vi "第一段判定.vi"(7 "Result":refnum<vi>, 10 "最大值判定":T1, 11 "XY曲线":cluster{"X":dbl[], "Y":dbl[]}[](array[cluster])) -> (2 "大小":i32, 3 "OK？":bool)   [LabVIEW 2020]
uses:
  Global_Variable/Global.vi
panel:
  in  "判定参数":T2
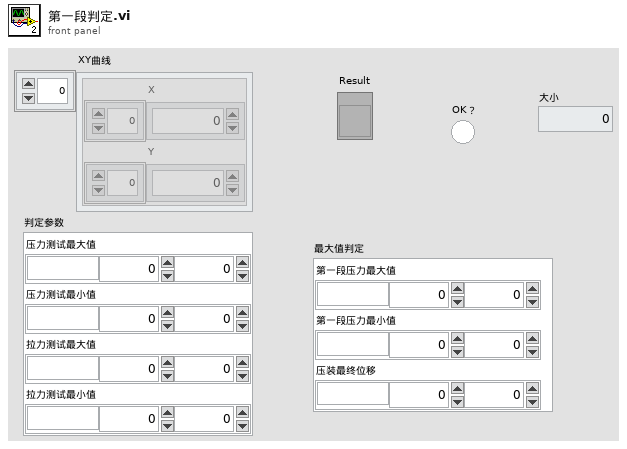
[diagram p1: front panel]
types:
  T1 = cluster{"第一段压力最大值":cluster{"单位":string, "下限":dbl, "上限":dbl}, "第一段压力最小值":cluster{"单位":string, "下限":dbl, "上限":dbl}, "压装最终位移":cluster{"单位":string, "下限":dbl, "上限":dbl}}
  T2 = cluster{"压力测试最大值":cluster{"单位":string, "下限":dbl, "上限":dbl}, "压力测试最小值":cluster{"单位":string, "下限":dbl, "上限":dbl}, "拉力测试最大值":cluster{"单位":string, "下限":dbl, "上限":dbl}, "拉力测试最小值":cluster{"单位":string, "下限":dbl, "上限":dbl}}
  T3 = cluster{"第一段判定框位移":cluster{"单位":string, "下限":dbl, "上限":dbl}, "第一段判定框压力":cluster{"单位":string, "下限":dbl, "上限":dbl}, "低二段判定框位移":cluster{"单位":string, "下限":dbl, "上限":dbl}, "第二段判定框压力":cluster{"单位":string, "下限":dbl, "上限":dbl}}
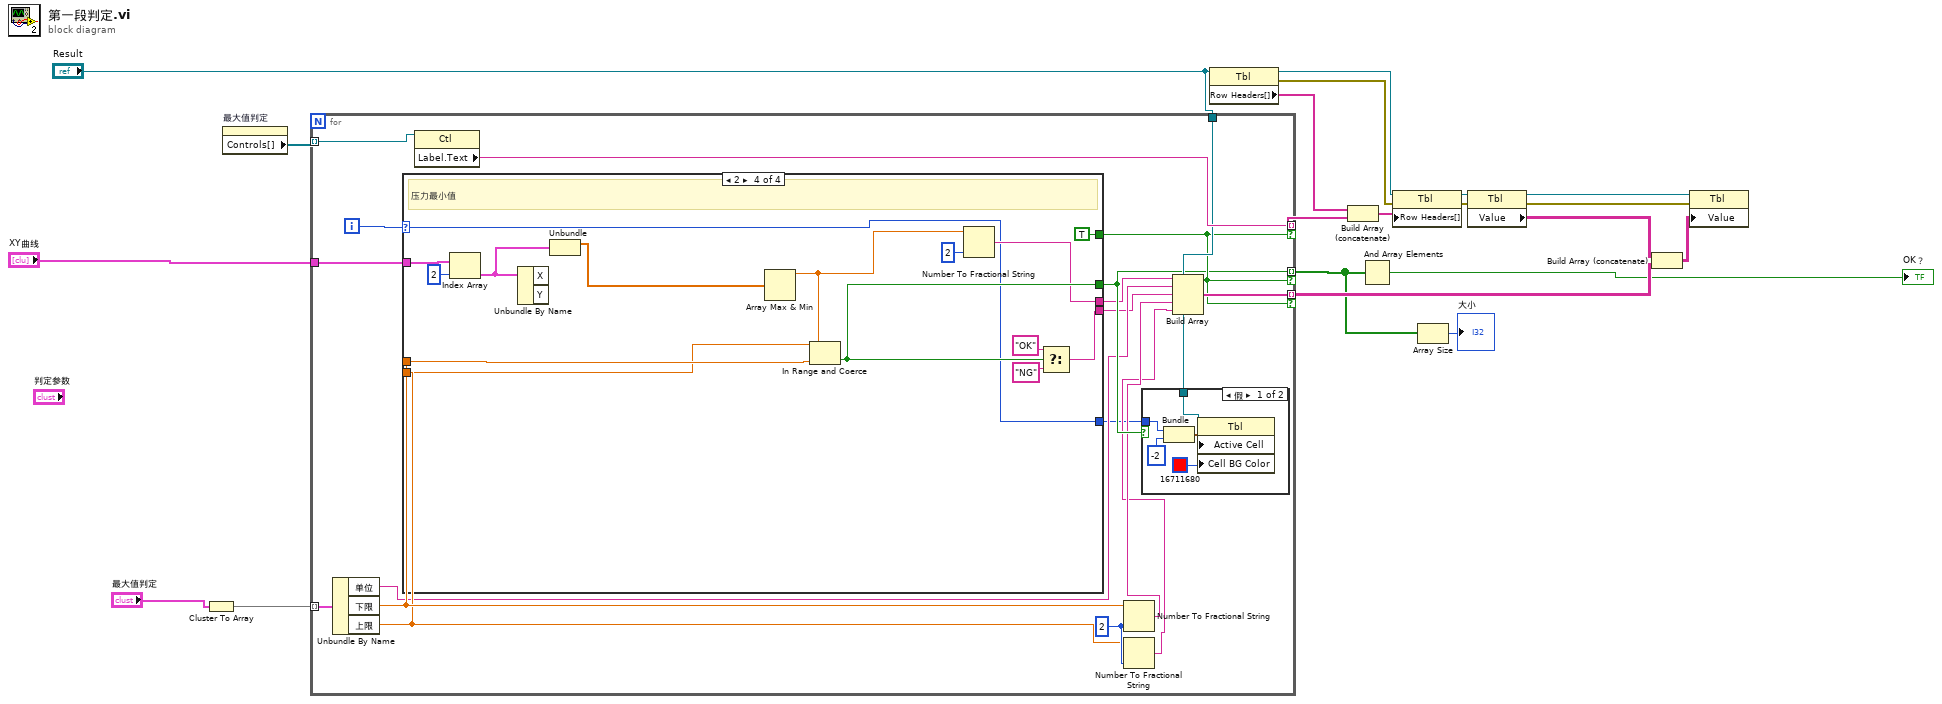
[diagram p0: block diagram]
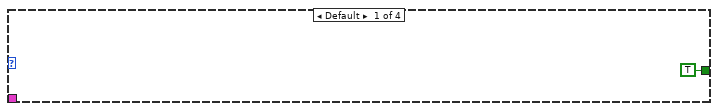
[diagram p3: hidden frame]
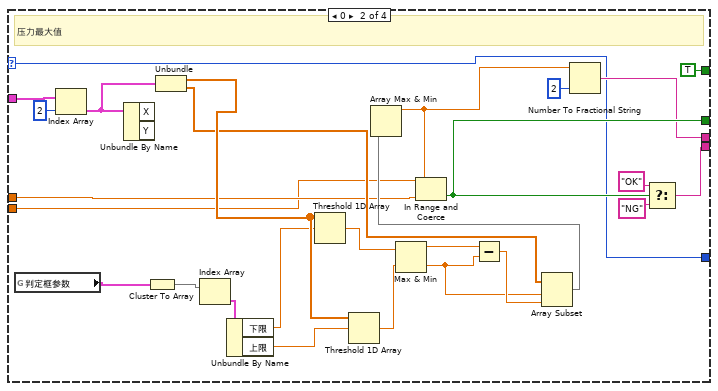
[diagram p4: hidden frame]
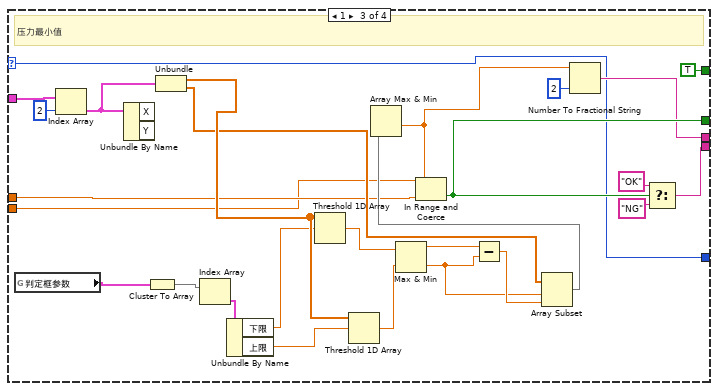
[diagram p5: hidden frame]
diagram:
  n1 = Cluster To Array(cluster="最大值判定") -> (array=w20:cluster{"单位":string, "下限":dbl, "上限":dbl}[])
  n2 = property on="最大值判定" class="Clust (严格)"() -> ("Controls[]"=w1:refnum<vi>[])  [unwired: 2 in, 2 out]
  n3 = for {
    tunnel: w20 -> [w38] mode=indexing
    tunnel: w1 -> [w36] mode=indexing
    tunnel: "XY曲线" -> [w35]
    tunnel: [w27] -> w3 mode=indexing if=w28
    tunnel: [w31] -> w7 mode=indexing if=w28
    tunnel: [w30] -> w9 mode=indexing if=w28
    tunnel: "Result" -> [w29]
    i -> [w37]
    w34 = i16 2 ("精度(6)")
    n4 = Unbundle By Name(w38) -> ("单位"=w25:string, "下限"=w33:dbl, "上限"=w32:dbl)
    n5 = case shown="2" w37 {
      selector: w37 -> [_ w52 w80 w103]
      tunnel: w35 -> [_ w71 w98 w113]
      tunnel: [_ w68 w95 w110] -> w24
      tunnel: [_ w67 w94 w109] -> w27
      tunnel: w33 -> [_ w51 w79 w102]
      tunnel: w32 -> [_ w50 w78 w101]
      tunnel: [TRUE TRUE TRUE TRUE] -> w28
      tunnel: [_ w53 w81 w104] -> w26
      tunnel: [_ w52 w80 w103] -> w21
      frame Default {
      }
      frame 0 {
        # "压力最大值"
        n6 = global read "Global.vi" "判定框参数"() -> (w45:T3)
        n7 = Index Array(array=w71, index=2 ("索引")) -> (element=w62:cluster{"X":dbl[], "Y":dbl[]})
        n8 = Unbundle By Name(w62) -> ()  [unwired: 2 out]
        n9 = Cluster To Array(cluster=w45) -> (array=w49:cluster{"单位":string, "下限":dbl, "上限":dbl}[])
        n10 = Unbundle(w62) -> ("X"=w61:dbl[], "Y"=w58:dbl[])
        n11 = Index Array(array=w49) -> (element=w48:cluster{"单位":string, "下限":dbl, "上限":dbl})  [unwired: 1 in]
        n12 = Unbundle By Name(w48) -> ("下限"=w47:dbl, "上限"=w46:dbl)
        n13 = Threshold 1D Array(2:w47, 3:w61) -> (0:w65:dbl)  [unwired: 1 in]
        n14 = Threshold 1D Array(2:w46, 3:w61) -> (0:w64:dbl)  [unwired: 1 in]
        n15 = Max & Min(x=w65, y=w64) -> (max(x,y)=w63:dbl, min(x,y)=w59:dbl)
        n16 = Subtract(x=w63, y=w59) -> (x-y=w60:dbl)
        n17 = Array Subset(array=w58, index=w59, length=w60) -> (w57:dbl[])
        n18 = Array Max & Min(array=w57) -> (max value=w54:dbl)  [unwired: 3 out]
        n19 = In Range and Coerce(upper limit=w50, x=w54, lower limit=w51) -> (In Range?=w67:bool)  [unwired: 1 out]
        n20 = Number To Fractional String(number=w54, precision (6)=i16 2 ("精度(6)")) -> (F-format string=w53:string)  [unwired: 2 in]
        n21 = Select(t="OK", s=w67, f="NG") -> (s? t:f=w68:string)
      }
      frame 1 {
        # "压力最小值"
        n22 = global read "Global.vi" "判定框参数"() -> (w73:T3)
        n23 = Index Array(array=w98, index=2 ("索引")) -> (element=w89:cluster{"X":dbl[], "Y":dbl[]})
        n24 = Unbundle By Name(w89) -> ()  [unwired: 2 out]
        n25 = Cluster To Array(cluster=w73) -> (array=w77:cluster{"单位":string, "下限":dbl, "上限":dbl}[])
        n26 = Unbundle(w89) -> ("X"=w88:dbl[], "Y"=w85:dbl[])
        n27 = Index Array(array=w77) -> (element=w76:cluster{"单位":string, "下限":dbl, "上限":dbl})  [unwired: 1 in]
        n28 = Unbundle By Name(w76) -> ("下限"=w75:dbl, "上限"=w74:dbl)
        n29 = Threshold 1D Array(2:w75, 3:w88) -> (0:w92:dbl)  [unwired: 1 in]
        n30 = Threshold 1D Array(2:w74, 3:w88) -> (0:w91:dbl)  [unwired: 1 in]
        n31 = Max & Min(x=w92, y=w91) -> (max(x,y)=w90:dbl, min(x,y)=w86:dbl)
        n32 = Subtract(x=w90, y=w86) -> (x-y=w87:dbl)
        n33 = Array Subset(array=w85, index=w86, length=w87) -> (w84:dbl[])
        n34 = Array Max & Min(array=w84) -> (min value=w72:dbl)  [unwired: 3 out]
        n35 = In Range and Coerce(upper limit=w78, x=w72, lower limit=w79) -> (In Range?=w94:bool)  [unwired: 1 out]
        n36 = Number To Fractional String(number=w72, precision (6)=i16 2 ("精度(6)")) -> (F-format string=w81:string)  [unwired: 2 in]
        n37 = Select(t="OK", s=w94, f="NG") -> (s? t:f=w95:string)
      }
      frame 2 {
        # "压力最小值"
        n38 = Index Array(array=w113, index=2 ("索引")) -> (element=w107:cluster{"X":dbl[], "Y":dbl[]})
        n39 = Unbundle By Name(w107) -> ()  [unwired: 2 out]
        n40 = Unbundle(w107) -> ("X"=w100:dbl[])  [unwired: 1 out]
        n41 = Array Max & Min(array=w100) -> (max value=w99:dbl)  [unwired: 3 out]
        n42 = In Range and Coerce(upper limit=w101, x=w99, lower limit=w102) -> (In Range?=w109:bool)  [unwired: 1 out]
        n43 = Number To Fractional String(number=w99, precision (6)=i16 2 ("精度(6)")) -> (F-format string=w104:string)  [unwired: 2 in]
        n44 = Select(t="OK", s=w109, f="NG") -> (s? t:f=w110:string)
      }
    }
    n45 = property class="Ctl"(reference=w36) -> ("Label.Text"=w30:string)  [unwired: 1 in, 2 out]
    n46 = Number To Fractional String(number=w33, precision (6)=w34) -> (F-format string=w23:string)  [unwired: 2 in]
    n47 = Number To Fractional String(number=w32, precision (6)=w34) -> (F-format string=w22:string)  [unwired: 2 in]
    n48 = case shown="假" w27 {
      tunnel: w29 -> [w43 _]
      tunnel: w21 -> [w39 _]
      frame False {
        n49 = Bundle(w39, -2) -> (w41:cluster{i32, i32})  [unwired: 1 in]
        n50 = property class="Tbl"(reference=w43, "Active Cell"=w41, "Cell BG Color"=u32 16711680 ("活动单元格:单元格背景色")) -> ()  [unwired: 1 in, 2 out]
      }
      frame True {
      }
    }
    n51 = Build Array(w26, w25, w24, w23, w22) -> (w31:string[])
  }
  n52 = property class="Tbl"(reference="Result") -> (reference out=w11:refnum<vi>, error out=w16:errorcluster, "Row Headers[]"=w8:string[])  [unwired: 1 in]
  n53 = Build Array (concatenate)(w8, w9) -> (w10:string[])
  n54 = And Array Elements(Boolean array=w3) -> (logical AND=→"OK？":bool)
  n55 = property class="Tbl"(reference=w11, error in=w16, "Row Headers[]"=w10) -> (reference out=w12:refnum<vi>, error out=w15:errorcluster)
  n56 = Array Size(array=w3) -> (size(s)=→"大小":i32)
  n57 = property class="Tbl"(reference=w12, error in=w15) -> (reference out=w13:refnum<vi>, error out=w14:errorcluster, "Value"=w17:string[][])
  n58 = Build Array (concatenate)(w17, w7) -> (w18:string[][])
  n59 = property class="Tbl"(reference=w13, error in=w14, "Value"=w18) -> ()  [unwired: 2 out]
